vi "dis_abs.vi"(1 "Numeric in":dbl, 2 "Numeric 3":dbl) -> (0 "distancia abs entre dos números":dbl)   [LabVIEW 2017]
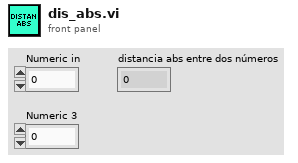
[diagram p1: front panel]
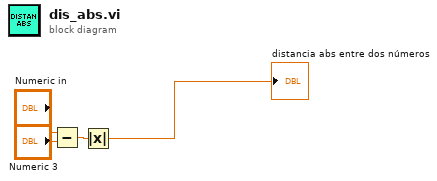
[diagram p0: block diagram]
diagram:
  n1 = Subtract(x="Numeric in", y="Numeric 3") -> (x-y=w2:dbl)
  n2 = Absolute Value(x=w2) -> (abs(x)=→"distancia abs entre dos números":dbl)
